vi "ShooterAngle.vi"(7 "Shooter Speed":T1(ring), 11 "Target Shooter Angle":T2(ring)) -> (2 "Shooter Angle Done":bool, 3 "Shooter Angle Good":bool)   [LabVIEW 2012]
uses:
  Robot Global Data.vi
  <vilib>/Rock Robotics/WPI/Solenoid/Deprecated/WPI_SolenoidSetBool.vi
panel:
  out "Returned Angle":u16
  in  "Shooter Up":bool
  in  "Target Angle":i32
  out "Shooter Angle State":u32
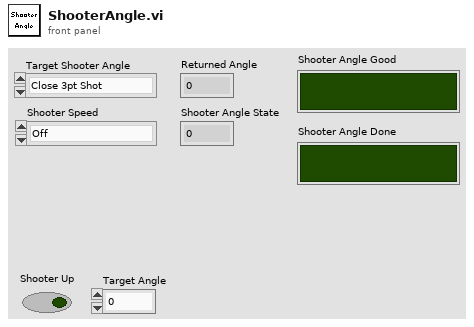
[diagram p1: front panel]
types:
  T1 = enum16{"Off", "Close Pyramid 3pt", "Far Pyramid 3pt", "Feeder Shot", "UD Far 3pt Shot"}
  T2 = enum16{"Close 3pt Shot", "Far 3pt Shot", "Feeding"}
  T3 = typedef "WPI_ServoDeviceRef.ctl" = cluster{"DeviceStatus":errorcluster, "Digital Module":T4, "PWM Channel":T5, "DeadBand":T6}
  T4 = typedef "FPGA_TypedefDigitalModule.ctl" = enum16{"Digital Module 1", "Digital Module 2"}
  T5 = typedef "FPGA_DIOPWMChannel.ctl" = enum8{"PWM 1", "PWM 2", "PWM 3", "PWM 4", "PWM 5", "PWM 6", "PWM 7", "PWM 8", "PWM 9", "PWM 10", "Invalid"}
  T6 = typedef "WPI_PWMDeadband.ctl" = cluster{"Name":string, "maxPositivePwm":i32, "minPositivePwm":i32, "centerPwm":i32, "maxNegativePwm":i32, "minNegativePwm":i32, "angularRange":u16}
  T7 = typedef "WPI_SolenoidDevRef.ctl" = cluster{"DevStatus":errorcluster, "Solenoid Module":T8, "Forward Solenoid Channel":T9, "Reverse Solenoid Channel":T9}
  T8 = typedef "FPGA_TypedefSolenoidModule.ctl" = enum16{"Solenoid Module 1", "Solenoid Module 2"}
  T9 = typedef "WPI_SolenoidChannel.ctl" = enum8{"Solenoid 1", "Solenoid 2", "Solenoid 3", "Solenoid 4", "Solenoid 5", "Solenoid 6", "Solenoid 7", "Solenoid 8", "Invalid"}
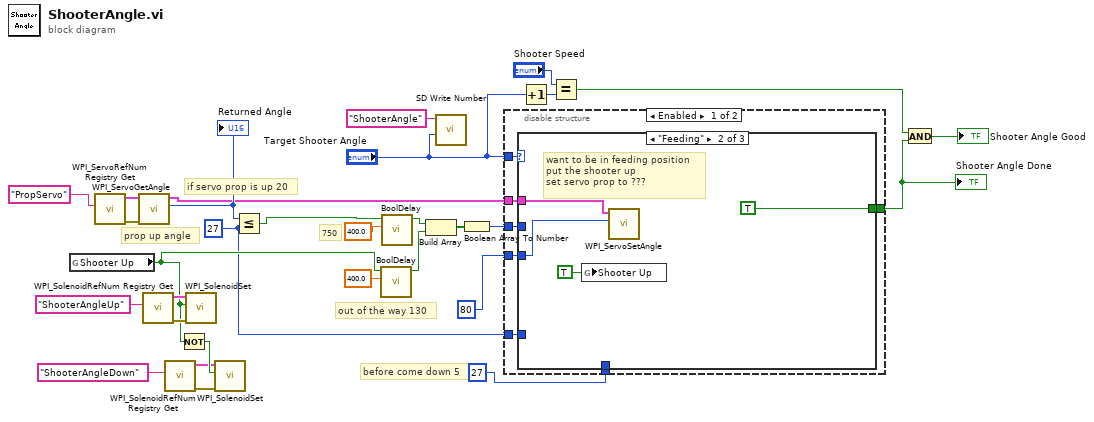
[diagram p0: block diagram]
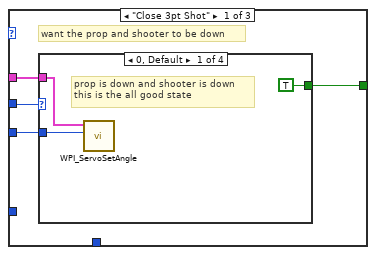
[diagram p2: hidden frame]
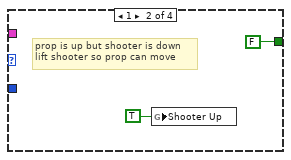
[diagram p3: hidden frame]
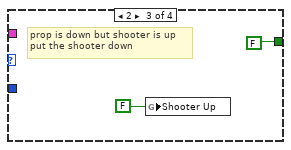
[diagram p4: hidden frame]
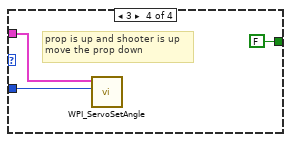
[diagram p5: hidden frame]
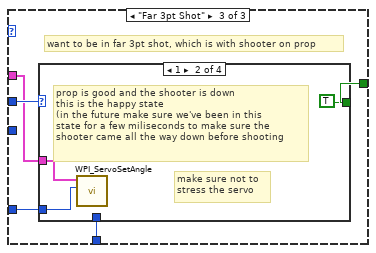
[diagram p6: hidden frame]
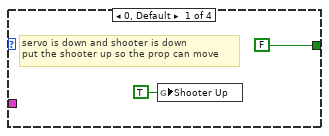
[diagram p7: hidden frame]
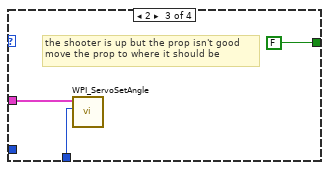
[diagram p8: hidden frame]
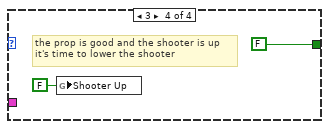
[diagram p9: hidden frame]
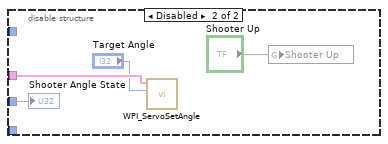
[diagram p10: hidden frame]
diagram:
  w1 = u16 27 ("y")
  # "750"
  # "before come down 5"
  # "prop up angle"
  # "out of the way 130"
  # "if servo prop is up 20"
  n1 = global read "Robot Global Data.vi" "Shooter Up"() -> (w10:bool)
  n2 = call <vilib>:"WPI_ServoRefNum Registry Get.vi"("refnum name"="PropServo") -> ("error out"=w21:errorcluster, "ServoDeviceRef"=w24:T3)  [unwired: 9 in]
  n3 = call <vilib>:"WPI_ServoGetAngle.vi"("ServoDeviceRef"=w24, "error in (no error)"=w21) -> ("ServoDeviceRef"=w19:T3, "Angle"=w20:u16)  [unwired: 6 in, 1 out]
  "Returned Angle" <- w20
  n4 = call <vilib>:"WPI_SolenoidRefNum Registry Get.vi"("refnum name"="ShooterAngleUp") -> ("error out"=w23:errorcluster, "SolenoidDevRef"=w29:T7)  [unwired: 9 in]
  n5 = call <vilib>:"WPI_SolenoidRefNum Registry Get.vi"("refnum name"="ShooterAngleDown") -> ("error out"=w22:errorcluster, "SolenoidDevRef"=w28:T7)  [unwired: 9 in]
  n6 = Not(x=w10) -> (.not. x?=w30:bool)
  n7 = call-poly <vilib>:"WPI_SolenoidSet.vi"("error in (no error)"=w23, "Value"=w10, "SolenoidDevRef"=w29) -> ()  [unwired: 7 in, 2 out]
  n8 = call-poly <vilib>:"WPI_SolenoidSet.vi"("error in (no error)"=w22, "Value"=w30, "SolenoidDevRef"=w28) -> ()  [unwired: 7 in, 2 out]
  n9 = Less Or Equal?(x=w20, y=w1) -> (x <= y?=w11:bool)
  n10 = call "BoolDelay.vi"("Delay"=400.0, "Input"=w10) -> ("Output"=w9:bool)  [unwired: 9 in]
  n11 = call "BoolDelay.vi"("Delay"=400.0, "Input"=w11) -> ("Output"=w12:bool)  [unwired: 9 in]
  n12 = Build Array(w12, w9) -> (w14:bool[])
  n13 = call <vilib>:"SD Write Number.vi"("Numeric"="Target Shooter Angle", "Name"="ShooterAngle") -> ()  [unwired: 8 in, 2 out]
  n14 = Boolean Array To Number(Boolean array=w14) -> (number=w13:u32)
  n15 = disable-structure shown="Enabled" {
    disable-tunnel: w19 -> [w37 w73]
    disable-tunnel: [w36 _] -> w5
    disable-tunnel: "Target Shooter Angle" -> [w35 _]
    disable-tunnel: w13 -> [w34 w74]
    disable-tunnel: 80 ("Angle") -> [w33 _]
    disable-tunnel: w1 -> [w32 _]
    disable-tunnel: 27 ("Angle") -> [w31 _]
    frame Enabled {
      n16 = case shown="\"Feeding\"" w35 {
        tunnel: w37 -> [w39 w54 w59]
        tunnel: w34 -> [w41 _ w60]
        tunnel: [w40 TRUE ("Shooter Up") w58] -> w36
        tunnel: w33 -> [w38 w52 _]
        tunnel: w32 -> [_ _ w57]
        tunnel: w31 -> [_ _ w56]
        frame "Close 3pt Shot" {
          # "want the prop and shooter to be down"
          n17 = case shown="0, Default" w41 {
            tunnel: [TRUE FALSE FALSE FALSE] -> w40
            tunnel: w39 -> [w42 _ _ w51]
            tunnel: w38 -> [w43 _ _ w49]
            frame 0, Default {
              # "prop is down and shooter is down\nthis is the all good state"
              n18 = call <vilib>:"WPI_ServoSetAngle.vi"("Angle"=w43, "ServoDeviceRef"=w42) -> ()  [unwired: 8 in, 2 out]
            }
            frame 1 {
              # "prop is up but shooter is down\nlift shooter so prop can move"
              n19 = global write "Robot Global Data.vi" "Shooter Up"(TRUE) -> ()
            }
            frame 2 {
              # "prop is down but shooter is up\nput the shooter down"
              n20 = global write "Robot Global Data.vi" "Shooter Up"(FALSE) -> ()
            }
            frame 3 {
              # "prop is up and shooter is up\nmove the prop down"
              n21 = call <vilib>:"WPI_ServoSetAngle.vi"("Angle"=w49, "ServoDeviceRef"=w51) -> ()  [unwired: 8 in, 2 out]
            }
          }
        }
        frame "Feeding" {
          # "want to be in feeding position\nput the shooter up\nset servo prop to ???"
          n22 = global write "Robot Global Data.vi" "Shooter Up"(TRUE ("Shooter Up")) -> ()
          n23 = call <vilib>:"WPI_ServoSetAngle.vi"("Angle"=w52, "ServoDeviceRef"=w54) -> ()  [unwired: 8 in, 2 out]
        }
        frame "Far 3pt Shot" {
          # "want to be in far 3pt shot, which is with shooter on prop"
          n24 = case shown="1" w60 {
            tunnel: w59 -> [_ w64 w68 _]
            tunnel: [FALSE TRUE FALSE FALSE] -> w58
            tunnel: w57 -> [_ w63 _ _]
            tunnel: w56 -> [_ _ w66 _]
            frame 0, Default {
              # "servo is down and shooter is down\nput the shooter up so the prop can move"
              n25 = global write "Robot Global Data.vi" "Shooter Up"(TRUE ("Shooter Up")) -> ()
            }
            frame 1 {
              # "make sure not to \nstress the servo"
              # "prop is good and the shooter is down\nthis is the happy state\n(in the future make sure we've been in this\nstate for a few miliseconds to make sure the \nshooter came all the way down before shooting"
              n26 = call <vilib>:"WPI_ServoSetAngle.vi"("Angle"=w63, "ServoDeviceRef"=w64) -> ()  [unwired: 8 in, 2 out]
            }
            frame 2 {
              # "the shooter is up but the prop isn't good\nmove the prop to where it should be"
              n27 = call <vilib>:"WPI_ServoSetAngle.vi"("Angle"=w66, "ServoDeviceRef"=w68) -> ()  [unwired: 8 in, 2 out]
            }
            frame 3 {
              # "the prop is good and the shooter is up\nit's time to lower the shooter"
              n28 = global write "Robot Global Data.vi" "Shooter Up"(FALSE ("Shooter Up")) -> ()
            }
          }
        }
      }
    }
    frame Disabled {
      n29 = call <vilib>:"WPI_ServoSetAngle.vi"("Angle"="Target Angle", "ServoDeviceRef"=w73) -> ()  [unwired: 8 in, 2 out]
      n30 = global write "Robot Global Data.vi" "Shooter Up"("Shooter Up") -> ()
      "Shooter Angle State" <- w74
    }
  }
  "Shooter Angle Done" <- w5
  n31 = Increment(x="Target Shooter Angle") -> (x+1=w15:T2)
  n32 = Equal?(x="Shooter Speed", y=w15) -> (x = y?=w16:bool)
  n33 = And(x=w16, y=w5) -> (x .and. y?=→"Shooter Angle Good":bool)
